vi "EvaluateHighRate.vi"(8 "error in (no error)":errorcluster, 9 "data in":T1, 10 "block number":u32) -> (0 "error out":errorcluster, 1 "data out":T1, 2 "complete":bool=TRUE)   [LabVIEW 2017, in "DataAccumulator.lvlib"]
uses:
  <vilib>/addons/InsightCM/Devices/Shared/Common/DataAccumulator/DataAccumulator.lvlib
  <vilib>/addons/InsightCM/Devices/Shared/Common/DataFlow/controls/Data.ctl
  <vilib>/addons/InsightCM/Utilities/DataAccessors/controls/wfmSGL_DVR.ctl
  <vilib>/addons/PointValueMap/controls/PointMap.ctl
  <vilib>/addons/InsightCM/Devices/Shared/Common/DataFlow/controls/Type.ctl
  <vilib>/addons/InsightCM/Devices/Shared/Common/DataAccumulator/controls/BlockParams.ctl
  <vilib>/addons/InsightCM/Devices/Shared/Common/DVRBuffer/controls/BufferLocation.ctl
  <vilib>/addons/PointValueMap/subVIs/Point_Read_double.vi
  <vilib>/addons/InsightCM/Devices/Shared/Common/DVRBuffer/DVRBuffer.lvlib
  <vilib>/addons/PointValueMap/PointValueMap.lvlib
  <vilib>/addons/InsightCM/Devices/Shared/Common/DataFlow/DataFlow.lvlib
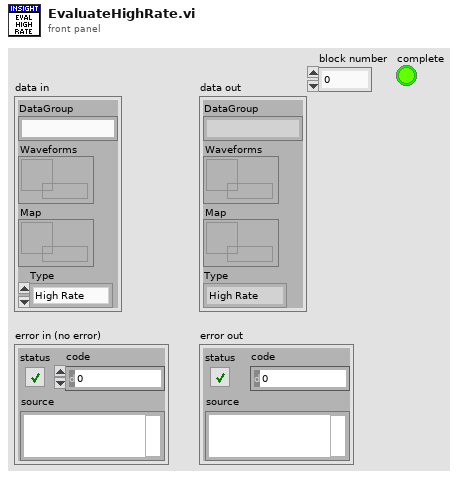
[diagram p1: front panel]
types:
  T1 = typedef "DataFlow.lvlib/Data.ctl" = cluster{"DataGroup":string, "Waveforms":T2, "Map":T3, "Type":T4}
  T2 = typedef "wfmSGL_DVR.ctl" = refnum<data-value>
  T3 = typedef "PointValueMap.lvlib/PointMap.ctl" = refnum<data-value>
  T4 = typedef "DataFlow.lvlib/Type.ctl" = enum16{"High Rate", "Low Rate", "Burst Mode"}
  T5 = typedef "DataAccumulator.lvlib/BlockParams.ctl" = cluster{"start block":T6, "stop block":T6, "BlockSizeSeconds":dbl}
  T6 = typedef "DVRBuffer.lvlib/BufferLocation.ctl" = cluster{"Block":u32, "Index":i32}
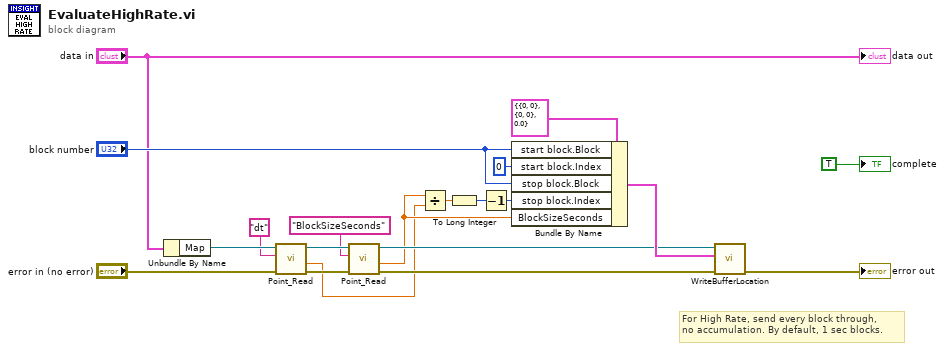
[diagram p0: block diagram]
diagram:
  # "For High Rate, send every block through,\nno accumulation. By default, 1 sec blocks."
  n1 = Unbundle By Name("data in") -> ("Map"=w11:T3)
  n2 = call-poly <vilib>:"Point_Read.vi"("Error In"="error in (no error)", "Tag"="dt", "Map"=w11) -> ("Error Out"=w14:errorcluster, "Value"=w6:dbl, "Map Out"=w12:T3)  [unwired: 3 in, 3 out]
  n3 = call-poly <vilib>:"Point_Read.vi"("Error In"=w14, "Tag"="BlockSizeSeconds", "Map"=w12) -> ("Error Out"=w13:errorcluster, "Value"=w7:dbl, "Map Out"=w10:T3)  [unwired: 3 in, 3 out]
  n4 = Divide(x=w7, y=w6) -> (x/y=w3:dbl)
  n5 = To Long Integer(number=w3) -> (32bit integer=w4:i32)
  n6 = Decrement(x=w4) -> (x-1=w5:i32)
  n7 = Bundle By Name(cluster=T5 {"start block"={"Block"=0, "Index"=0}, "stop block"={"Block"=0, "Index"=0}, "BlockSizeSeconds"=0.0} ("BlockParams"), "start block.Block"="block number", "start block.Index"=0, "stop block.Block"="block number", "stop block.Index"=w5, "BlockSizeSeconds"=w7) -> (w16:T5)
  n8 = call <vilib>:"WriteBufferLocation.vi"("error in (no error)"=w13, "block params"=w16, "map in"=w10) -> ("error out"=→"error out":errorcluster)  [unwired: 7 in, 1 out]
  "data out" <- "data in"
  "complete" <- TRUE
